vi "Calibrate.vi"(8 "error in (no error)":errorcluster, 11 "Instrument in":refnum<class "DMM.NI.lvclass">) -> (0 "error out":errorcluster, 1 "Success?":bool, 2 "Result":variant, 3 "Instrument out":refnum<class "DMM.NI.lvclass">)   [LabVIEW 2020, in "NI DMM Driver.lvlib" / "DMM.NI.lvclass"]
doc: "Calibrate the instrument if supported. The calibration result is returned in a variant.\n\nThis implementation performs a NI DMM self calibration if supported."
uses:
  DMM.NI.lvclass
  <instrlib>/niDMM/nidmm.llb/niDMM Cal Type.ctl
  <vilib>/Utility/miscctls.llb/LVDateTimeRec.ctl
  NI DMM Calibration Data/NI DMM Calibration Data.lvclass
  PPL/HDH.Actor Framework.Core.Instrument Driver.lvlibp/Instrument Driver/Instrument Driver.lvclass
  C:/Current projects/WS/PPL/HDH.Driver.DMM.lvlibp/DMM Driver.lvclass
  C:/Current projects/WS/PPL/HDH.Actor Framework.Core.Instrument Driver.lvlibp/Instrument Driver/Instrument Driver.lvclass
  C:/Current projects/WS/LV32.2020.HDH.Driver.DMM/DMM.NI/NI/DMM.NI.lvclass
  C:/Current projects/WS/PPL/HDH.Data.Generic.lvlibp/Data.lvclass
  C:/Users/Henri/OneDrive/LabVIEW/Instruments/DMM/NI DMM Driver/Data/NI DMM Calibration Data/NI DMM Calibration Data.lvclass
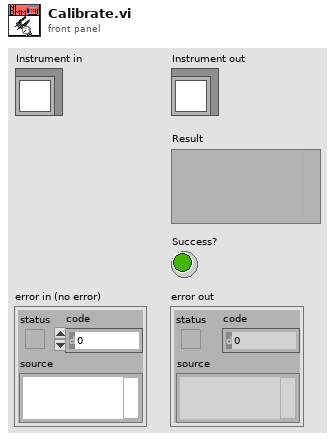
[diagram p1: front panel]
types:
  T1 = typedef "LVDateTimeRec.ctl" = cluster{"fractional second":dbl, "second":i32, "minute":i32, "hour":i32, "day of month":i32, "month":i32, "year":i32, "day of week":i32, "day of year":i32, "DST":i32}
  T2 = typedef "niDMM Cal Type.ctl" = enum16{"Internal", "External"}
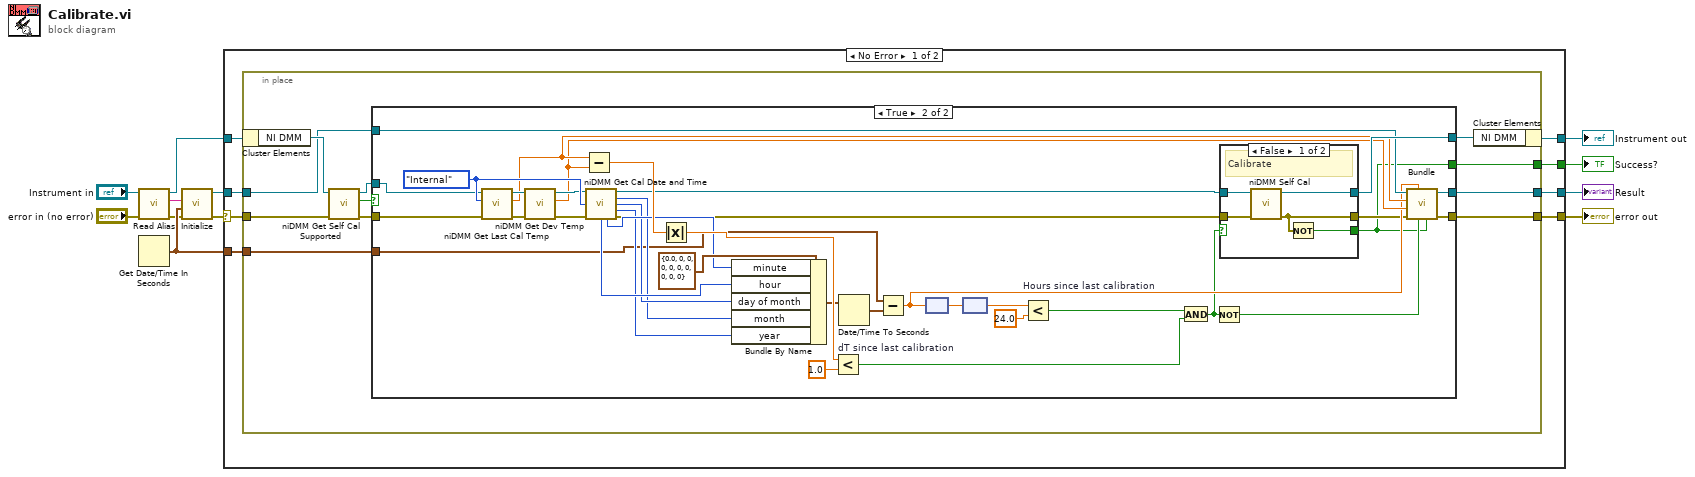
[diagram p0: block diagram]
diagram:
  n1 = call "Read Alias.vi"("error in (no error)"="error in (no error)", "Instrument in"="Instrument in") -> ("error out"=w4:errorcluster, "Alias"=w5:string, "Instrument out"=w8:refnum<class "DMM.NI.lvclass">)  [unwired: 7 in]
  n2 = Get Date/Time In Seconds() -> (seconds since 1Jan1904=w6:timestamp)
  n3 = call "Initialize.vi"("error in (no error)"=w4, "Time"=w6, "Alias"=w5) -> ("error out"=w3:errorcluster, "NI DMM Calibration Data out"=w2:refnum<class "NI DMM Calibration Data.lvclass">)  [unwired: 7 in]
  n4 = case shown="No Error" w3 {
    selector: w3 -> [w17 w83]
    tunnel: w8 -> [w20 w82]
    tunnel: [w19 w82] -> w12
    tunnel: [w18 _] -> w11
    tunnel: [w16 w83] -> w10
    tunnel: w6 -> [w15 _]
    tunnel: w2 -> [w13 w81]
    tunnel: [w14 w81] -> w1
    frame No Error {
      n5 = in-place {
        in-place-border: [w27] -> w18
        in-place-border: w17 -> [w26]
        in-place-border: [w25] -> w16
        in-place-border: w15 -> [w23]
        in-place-border: [w22] -> w14
        in-place-border: w13 -> [w21]
        n6 = in-place-cluster #1(w20) -> ("NI DMM"=w31:refnum<k15>)
        n7 = call <instrlib>:"niDMM Get Self Cal Supported.vi"("error in (no error)"=w26, "instrument handle"=w31) -> ("error out"=w24:errorcluster, "Self Cal Supported?"=w30:bool, "instrument handle out"=w28:refnum<k15>)  [unwired: 7 in]
        n8 = case shown="True" w30 {
          selector: w30 -> [w34 _]
          tunnel: [w35 w49] -> w29
          tunnel: w28 -> [w35 w71]
          tunnel: [w34 w36] -> w27
          tunnel: [w33 w40] -> w25
          tunnel: w24 -> [w33 w69]
          tunnel: w23 -> [_ w47]
          tunnel: [w32 w39] -> w22
          tunnel: w21 -> [w32 w46]
          frame False {
          }
          frame True {
            w72 = niDMM_Cal_Type."Internal" ("Cal Type")
            n9 = call <instrlib>:"niDMM Get Last Cal Temp.vi"("error in (no error)"=w69, "Cal Type"=w72, "instrument handle"=w71) -> ("error out"=w68:errorcluster, "Temperature"=w45:dbl, "instrument handle out"=w70:refnum<k15>)  [unwired: 6 in]
            n10 = call <instrlib>:"niDMM Get Dev Temp.vi"("error in (no error)"=w68, "instrument handle"=w70) -> ("error out"=w43:errorcluster, "Temperature"=w44:dbl, "instrument handle out"=w65:refnum<k15>)  [unwired: 7 in]
            n11 = Subtract(x=w45, y=w44) -> (x-y=w67:dbl)
            n12 = call <instrlib>:"niDMM Get Cal Date and Time.vi"("instrument handle"=w65, "Cal Type"=w72, "error in (no error)"=w43) -> ("instrument handle out"=w50:refnum<k15>, "Month"=w59:i32, "Day"=w60:i32, "Year"=w61:i32, "Hour"=w62:i32, "Minute"=w63:i32, "error out"=w51:errorcluster)  [unwired: 6 in]
            n13 = Absolute Value(x=w67) -> (abs(x)=w66:dbl)
            n14 = Bundle By Name(cluster=T1 {"fractional second"=0.0, "second"=0, "minute"=0, "hour"=0, "day of month"=0, "month"=0, "year"=0, "day of week"=0, "day of year"=0, "DST"=0} ("date time rec"), "minute"=w63, "hour"=w62, "day of month"=w60, "month"=w59, "year"=w61) -> (w58:T1)
            n15 = Less? "dT since last calibration"(x=w66, y=1.0) -> (x < y?=w52:bool)
            n16 = Date/Time To Seconds(2:w58) -> (0:w57:timestamp)  [unwired: 1 in]
            n17 = Subtract(x=w47, y=w57) -> (x-y=w42:dbl)
            n18 = node(w42) -> (w56:dbl[unit])
            n19 = node(w56) -> (w55:dbl)
            n20 = Less? "Hours since last calibration"(x=w55, y=24.0) -> (x < y?=w53:bool)
            n21 = And(x=w53, y=w52) -> (x .and. y?=w38:bool)
            n22 = Not(x=w38) -> (.not. x?=w37:bool)
            n23 = case shown="False" w38 {
              selector: w38 -> [_ w78]
              tunnel: [w74 w80] -> w41
              tunnel: w51 -> [w76 w80]
              tunnel: w50 -> [w77 w79]
              tunnel: [w73 w79] -> w49
              tunnel: [w75 w78] -> w36
              frame False {
                # "Calibrate"
                n24 = call <instrlib>:"niDMM Self Cal.vi"("error in (no error)"=w76, "instrument handle"=w77) -> ("error out"=w74:errorcluster, "instrument handle out"=w73:refnum<k15>)  [unwired: 8 in]
                n25 = Not(x=w74) -> (.not. x?=w75:bool)
              }
              frame True {
                # "Calibration not needed"
              }
            }
            n26 = call "Bundle.vi"("Success?"=w36, "Calibration Needed?"=w37, "Hours since last Cal"=w42, "error in (no error)"=w41, "Current T"=w44, "Last Cal T"=w45, "NI DMM Calibration Data in"=w46) -> ("error out"=w40:errorcluster, "NI DMM Calibration Data out"=w39:refnum<class "NI DMM Calibration Data.lvclass">)  [unwired: 3 in]
          }
        }
        n27 = in-place-cluster #1("NI DMM"=w29) -> (w19:refnum<class "DMM.NI.lvclass">)
      }
    }
    frame Error {
    }
  }
  "error out" <- w10
  "Instrument out" <- w12
  "Success?" <- w11
  "Result" <- w1
